vi "Task Awaiter.vi"(8 "error in (no error)":errorcluster, 10 "Timeout":i32=-1, 11 "Task":refnum<k24>) -> (0 "error out":errorcluster, 2 "Timeout":bool, 3 "Task":refnum<k24>)   [LabVIEW 2024, in "WebView.lvclass"]
uses:
  WebView.lvclass
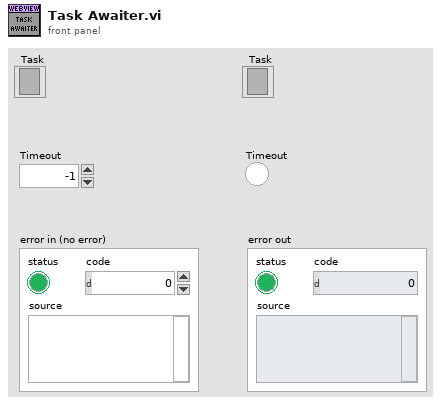
[diagram p1: front panel]
types:
  T1 = enum32{"Created", "WaitingForActivation", "WaitingToRun", "Running", "WaitingForChildrenToComplete", "RanToCompletion", "Canceled", "Faulted"}
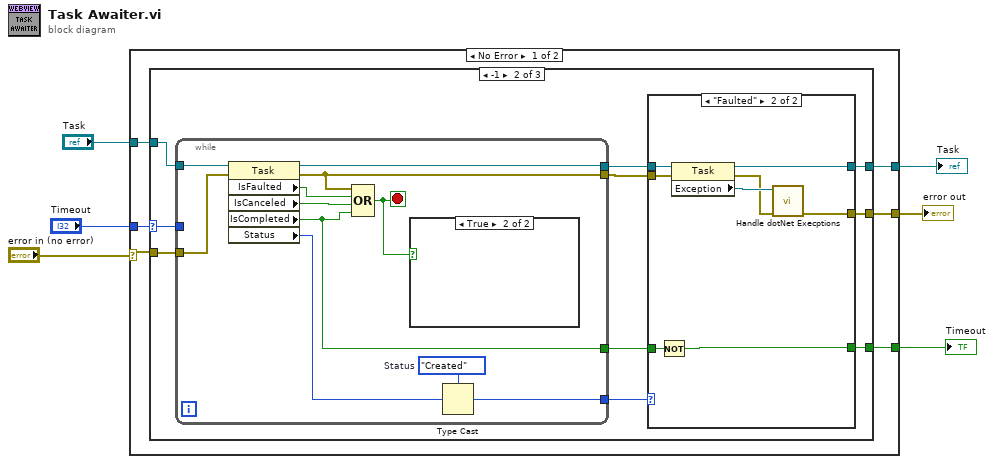
[diagram p0: block diagram]
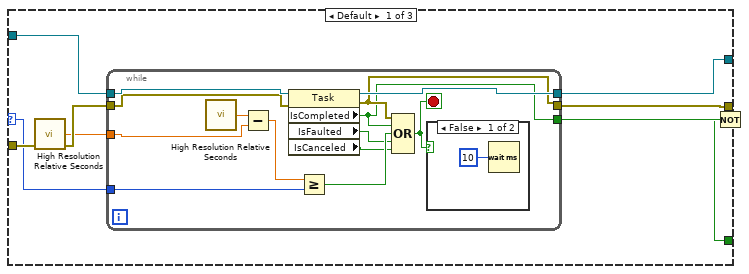
[diagram p2: hidden frame]
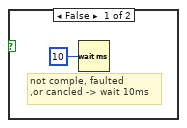
[diagram p5: hidden frame]
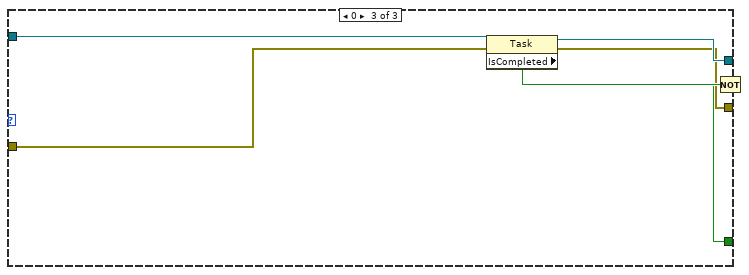
[diagram p6: hidden frame]
diagram:
  n1 = case shown="No Error" "error in (no error)" {
    selector: "error in (no error)" -> [w11 w75]
    tunnel: "Task" -> [w12 w74]
    tunnel: "Timeout" -> [w10 _]
    tunnel: [w9 w75] -> w3
    tunnel: [w8 w74] -> w2
    tunnel: [w7 _] -> w1
    frame No Error {
      n2 = case shown="-1" w10 {
        selector: w10 -> [w17 w42 _]
        tunnel: w12 -> [w20 w44 w73]
        tunnel: w11 -> [w19 w43 w72]
        tunnel: [w18 w38 w71] -> w8
        tunnel: [w16 w36 w68] -> w9
        tunnel: [w13 w40 w69] -> w7
        frame Default {
          n3 = call <vilib>:"High Resolution Relative Seconds.vi"() -> ("relative seconds"=w15:dbl)
          n4 = while {
            tunnel: w20 -> [w33]
            tunnel: w19 -> [w32]
            tunnel: [w31] -> w18
            tunnel: w15 -> [w29]
            tunnel: w17 -> [w27]
            tunnel: [w25] -> w16
            tunnel: [w24] -> w14
            stop <- w21 stop-if-true
            n5 = call <vilib>:"High Resolution Relative Seconds.vi"() -> ("relative seconds"=w30:dbl)
            n6 = Subtract(x=w30, y=w29) -> (x-y=w28:dbl)
            n7 = property class="Task"(reference=w33, error in=w32) -> (reference out=w31:refnum<k24>, error out=w25:errorcluster, "IsCompleted"=w24:bool, "IsFaulted"=w23:bool, "IsCanceled"=w22:bool)
            n8 = Greater Or Equal?(x=w28, y=w27) -> (x >= y?=w26:bool)
            n9 = Compound Arithmetic op=OR(w25, w24, w26, w23, w22) -> (w21:bool)
            n10 = case shown="False" w21 {
              frame False {
                n11 = Wait (ms)(milliseconds to wait=u32 10) -> ()  [unwired: 1 out]
              }
              frame True {
              }
            }
          }
          n12 = Not(x=w14) -> (.not. x?=w13:bool)
        }
        frame -1 {
          n13 = while {
            tunnel: w44 -> [w66]
            tunnel: w43 -> [w65]
            tunnel: [w64] -> w39
            tunnel: w42 -> [_]
            tunnel: [w63] -> w37
            tunnel: [w59] -> w41
            tunnel: [w57] -> w35
            stop <- w61 stop-if-true
            w56 = T1."Created"  # Status
            n14 = property class="Task"(reference=w66, error in=w65) -> (reference out=w64:refnum<k24>, error out=w63:errorcluster, "IsFaulted"=w60:bool, "IsCanceled"=w62:bool, "IsCompleted"=w59:bool, "Status"=w58:i32)
            n15 = Compound Arithmetic op=OR(w63, w60, w62, w59) -> (w61:bool)
            n16 = case shown="True" w61 {
              frame False {
                # "not comple, faulted\n,or cancled -> wait 10ms"
                n17 = Wait (ms)(milliseconds to wait=u32 10) -> ()  [unwired: 1 out]
              }
              frame True {
              }
            }
            n18 = Type Cast(type=w56, x=w58) -> (*(type *) &x=w57:T1)
          }
          n19 = case shown="\"Faulted\"" w35 {
            tunnel: w41 -> [w45 w55]
            tunnel: [w45 w54] -> w40
            tunnel: w39 -> [w47 w52]
            tunnel: [w47 w51] -> w38
            tunnel: w37 -> [w46 w50]
            tunnel: [w46 w49] -> w36
            frame Default {
            }
            frame "Faulted" {
              n20 = Not(x=w55) -> (.not. x?=w54:bool)
              n21 = property class="Task"(reference=w52, error in=w50) -> (reference out=w51:refnum<k24>, error out=w48:errorcluster, "Exception"=w53:refnum<k24>)
              n22 = call "Handle dotNet Execptions.vi"("error in (no error)"=w48, ".NET Refnum in"=w53) -> ("error out"=w49:errorcluster)  [unwired: 9 in]
            }
          }
        }
        frame 0 {
          n23 = property class="Task"(reference=w73, error in=w72) -> (reference out=w71:refnum<k24>, error out=w68:errorcluster, "IsCompleted"=w70:bool)
          n24 = Not(x=w70) -> (.not. x?=w69:bool)
        }
      }
    }
    frame Error {
    }
  }
  "error out" <- w3
  "Task" <- w2
  "Timeout" <- w1
